vi "Disconnect.vi"(8 "error in (no error)":errorcluster, 11 "Potentiostat Galvanostat in":refnum<class "Potentiostat Galvanostat.lvclass">) -> (0 "error out":errorcluster)   [LabVIEW 2018, in "Potentiostat Galvanostat.lvclass"]
uses:
  Potentiostat Galvanostat.lvclass
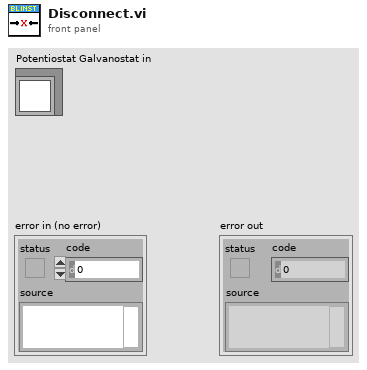
[diagram p1: front panel]
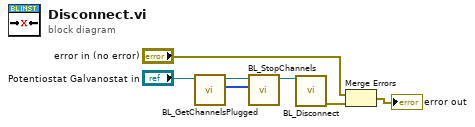
[diagram p0: block diagram]
diagram:
  n1 = call-dynamic "BL_GetChannelsPlugged .vi"("Potentiostat Galvanostat in"="Potentiostat Galvanostat in") -> ("Plugged Channels"=w6:u8[], "Potentiostat Galvanostat out"=w5:refnum<class "Potentiostat Galvanostat.lvclass">)  [unwired: 8 in, 1 out]
  n2 = call-dynamic "BL_StopChannels.vi"("Channles"=w6, "Potentiostat Galvanostat in"=w5) -> ("Potentiostat Galvanostat out"=w4:refnum<class "Potentiostat Galvanostat.lvclass">)  [unwired: 6 in, 3 out]
  n3 = call "BL_Disconnect.vi"("Potentiostat Galvanostat in"=w4) -> ("error out"=w3:errorcluster)  [unwired: 9 in, 1 out]
  n4 = Merge Errors("error in (no error)", w3) -> (→"error out":errorcluster)
